vi "Cliente.vi"(8 "error in (no error)":errorcluster, 9 "tmsg":i32, 10 "port":i32, 11 "addr_srv":string) -> (0 "error out":errorcluster, 3 "Cliente out":refnum<class "Cliente.lvclass">)   [LabVIEW 2016, in "Cliente.lvclass"]
uses:
  Cliente.lvclass
  Mensagem.lvclass/Mensagem.ctl
  Cliente.lvclass/Cliente.ctl
  Mensagem.lvclass
panel:
  out "local port":u16
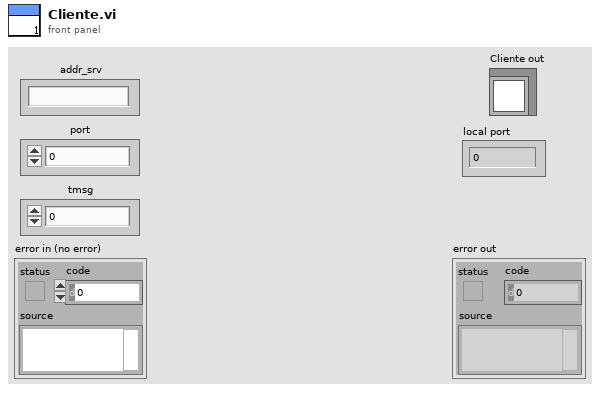
[diagram p1: front panel]
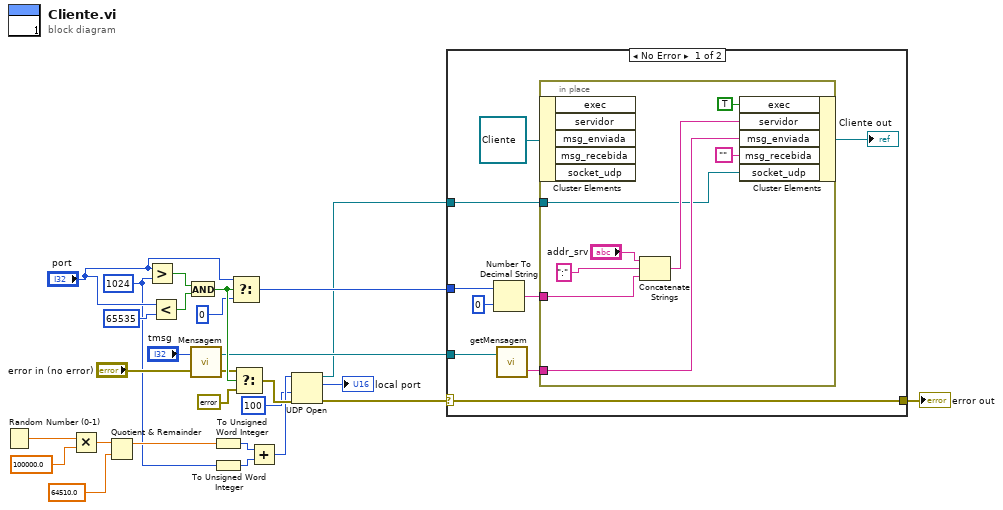
[diagram p0: block diagram]
diagram:
  w6 = 1024
  n1 = Random Number (0-1)() -> (number: 0 to 1=w13:dbl)
  n2 = Multiply(x=w13, y=100000.0) -> (x*y=w8:dbl)
  n3 = Quotient & Remainder(x=w8, y=64510.0) -> (x-y*floor(x/y)=w7:dbl)  [unwired: 1 out]
  n4 = Greater?(x="port", y=w6) -> (0:w22:bool)
  n5 = Less?(x="port", y=65535) -> (x < y?=w23:bool)
  n6 = And(x=w22, y=w23) -> (x .and. y?=w20:bool)
  n7 = call "Mensagem.vi"("error in (no error)"="error in (no error)", "tamanho"="tmsg") -> ("error IO"=w19:errorcluster, "Mensagem"=w16:refnum<class "Mensagem.lvclass">)
  n8 = To Unsigned Word Integer(number=w7) -> (unsigned 16bit integer=w11:u16)
  n9 = To Unsigned Word Integer(number=w6) -> (unsigned 16bit integer=w10:u16)
  n10 = Select(t="port", s=w20, f=0 ("width (-)")) -> (s? t:f=w17:i32)
  n11 = Select(t=w19, s=w20, f=errorcluster {"status"=TRUE, "code"=-1, "source"="Numero de porta deve está entre 1024 e 65535!!!"}) -> (s? t:f=w14:errorcluster)
  n12 = Add(x=w11, y=w10) -> (x+y=w9:u16)
  n13 = UDP Open(8:w14, 9:100 ("timeout ms (25000)"), 11:w9) -> (port=w3:refnum<k16>, 0:w2:errorcluster, 2:→"local port":u16)  [unwired: 2 in]
  n14 = case shown="No Error" w2 {
    selector: w2 -> [w34 w45]
    tunnel: [w34 w45] -> w27
    tunnel: w17 -> [w30 _]
    tunnel: w16 -> [w29 _]
    tunnel: w3 -> [w28 _]
    frame No Error {
      n15 = Number To Decimal String(number=w30, width (-)=i16 0) -> (decimal integer string=w33:string)
      n16 = call "getMensagem.vi"("Mensagem in"=w29) -> ("mensagem"=w31:string)  [unwired: 1 in, 1 out]
      n17 = in-place {
        in-place-border: w31 -> [w43]
        in-place-border: w33 -> [w38]
        in-place-border: w28 -> [w37]
        n18 = in-place-cluster #1(refnum<class "Cliente.lvclass"> refnum ("Cliente.lvclass")) -> ()  [unwired: 5 out]
        n19 = Concatenate Strings("addr_srv", ":", w38) -> (w40:string)
        n20 = in-place-cluster #1("exec"=TRUE, "servidor"=w40, "msg_enviada"=w43, "msg_recebida"="", "socket_udp"=w37) -> (→"Cliente out":refnum<class "Cliente.lvclass">)
      }
    }
    frame Error {
    }
  }
  "error out" <- w27
